vi "Update Controller State.vi"(8 "error in (no error)":errorcluster, 11 "Car Wash Controller in":refnum<class "Car Wash Controller.lvclass">) -> (0 "error out":errorcluster, 3 "Car Wash Controller out":refnum<class "Car Wash Controller.lvclass">)   [LabVIEW 2019, in "Car Wash Controller.lvlib" / "Car Wash Controller.lvclass"]
uses:
  Car Wash Controller.lvclass
  <vilib>/ActorFramework/Actor/Actor.lvclass
  Sim Configuration Database Actor/Sim Configuration Database Actor Messages/Read Record Msg/Read Record Msg.lvclass
  Sim Configuration Database Actor/Sim Configuration Database Actor Messages/Select DB Msg/Select DB Msg.lvclass
  Sim Configuration Database Actor/Sim Configuration Database Actor Messages/Write Record Msg/Write Record Msg.lvclass
  Sim Configuration Database Actor/Sim Configuration Database Actor/Database Type.ctl
  Sim Configuration Database Actor/Sim Configuration Database Actor/Sim Configuration Database Actor.lvclass
  Sim Entry Console Actor/Sim Entry Console Actor Messages/Enable Wash Steps Msg/Enable Wash Steps Msg.lvclass
  Sim Entry Console Actor/Sim Entry Console Actor Messages/Enable Start Msg/Enable Start Msg.lvclass
  Sim Wash Display Console/Sim Wash Display Console Messages/Write Remaining timing Msg/Write Remaining timing Msg.lvclass
  Sim Wash Display Console/Sim Wash Display Console Messages/Write Vehicle Out of Position Msg/Write Vehicle Out of Position Msg.lvclass
  Sim Wash Display Console/Sim Wash Display Console Messages/Write Wash Step Indicator Msg/Write Wash Step Indicator Msg.lvclass
  Sim Wash Display Console/Sim Wash Display Console Messages/Write Wash Entry Msg/Write Wash Entry Msg.lvclass
  Wash Steps.ctl
  Vehicle Position Simulation Actor/Vehicle Position Simulation Actor Messages/Write Vehicle Position Msg/Write Vehicle Position Msg.lvclass
  <vilib>/ActorFramework/Message Enqueuer/Message Enqueuer.lvclass
  Car Wash Controller Messages/Set Vehicle Position Msg/Set Vehicle Position Msg.lvclass
  Car Wash Controller Messages/Set Entry Position Msg/Set Entry Position Msg.lvclass
  Vehicle Position Simulation Actor/Car Wash Controller/Station -Enum.ctl
  Vehicle Position Simulation Actor/Car Wash Controller/Vehicle Position Simulation Actor.lvclass
  Car Wash Controller Messages/Set State Msg/Set State Msg.lvclass
  States -Enum.ctl
  C:/Program Files (x86)/National Instruments/LabVIEW 2019/vi.lib/ActorFramework/Actor/Actor.lvclass
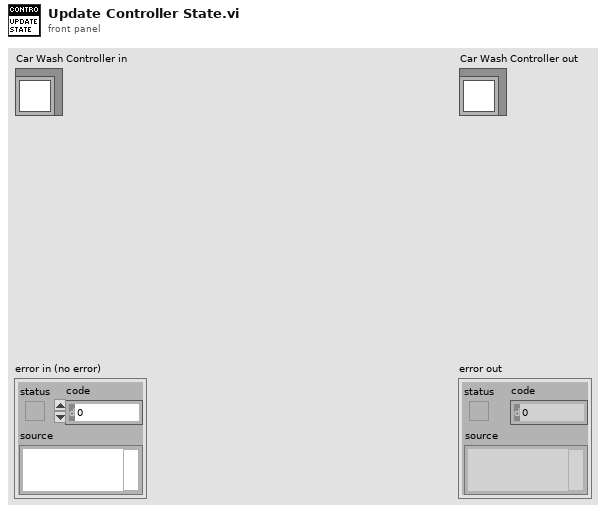
[diagram p1: front panel]
types:
  T1 = typedef "Car Wash Controller.lvlib/Car Wash Controller.lvclass/Wash Steps.ctl" = cluster{"Under Body Wash":bool, "Bug Remover":bool, "Pre-Soak":bool, "High Pressure Wash (Default)":bool, "Low Pressure Wax":bool, "Spot Free Rinse":bool, "Tire Shine Foam":bool, "Air Dry":bool}
  T2 = enum8{"Enabled", "Disabled", "Disabled and Grayed Out"}
  T3 = typedef "Sim Configuration Database Actor.lvlib/Sim Configuration Database Actor.lvclass/Database Type.ctl" = enum16{"Default", "Client"}
  T4 = typedef "Car Wash Controller.lvlib/Car Wash Controller.lvclass/States -Enum.ctl" = enum16{"Inital", "Wait for Start", "Start", "Wait for Vehicle Position", "Wash Step Execution", "Wash Step/Cycle Completion", "Wash Exit", "Wash Abort/Terminate State"}
  T5 = typedef "Vehicle Position Sinmulation Actor.lvlib/Vehicle Position Simulation Actor.lvclass/Station -Enum.ctl" = enum16{"Entry", "Station1", "Station2", "Station3", "Exit"}
  T6 = typedef "Sim Configuration Database Actor.lvlib/Sim Configuration Database Actor.lvclass/Record.ctl" = cluster{"Wash Step":string, "Step Duration":dbl, "Station":T5}
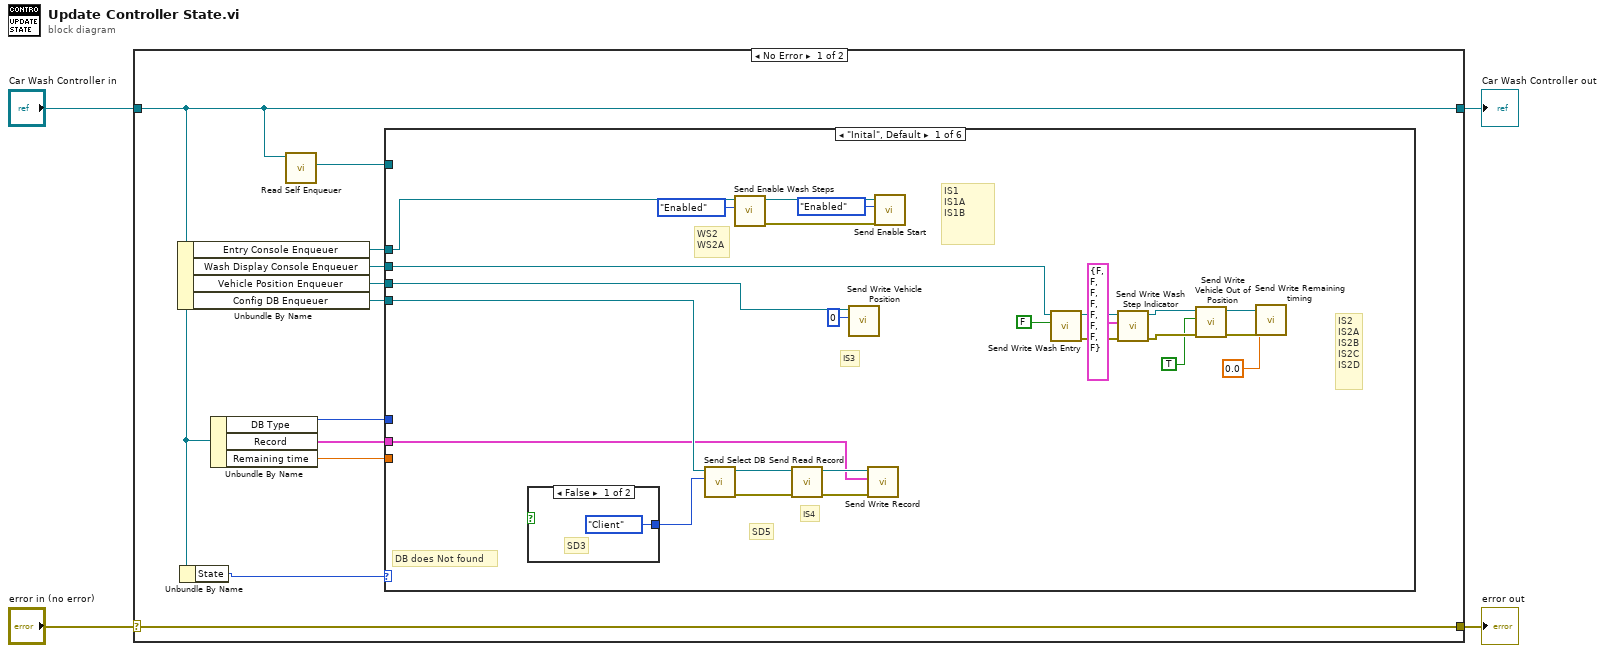
[diagram p0: block diagram]
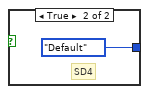
[diagram p2: hidden frame]
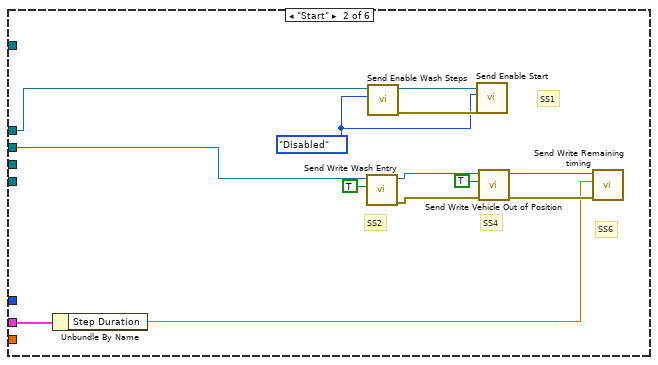
[diagram p3: hidden frame]
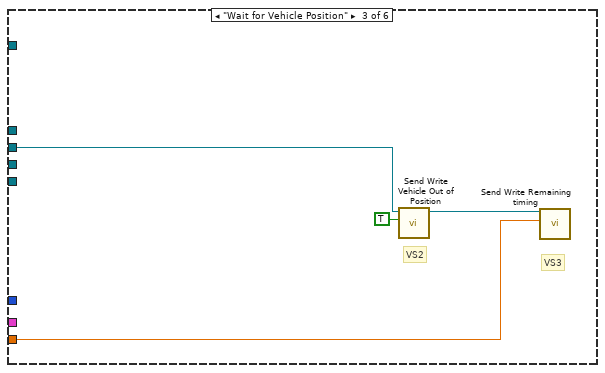
[diagram p4: hidden frame]
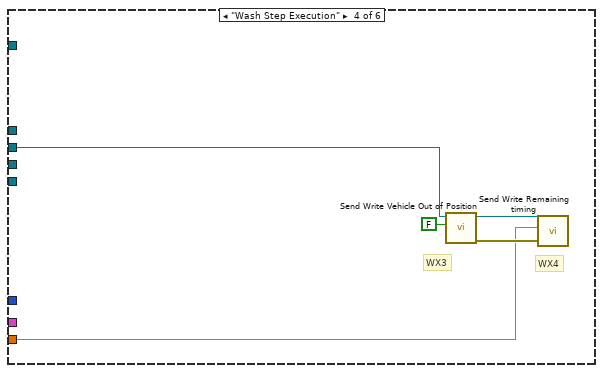
[diagram p5: hidden frame]
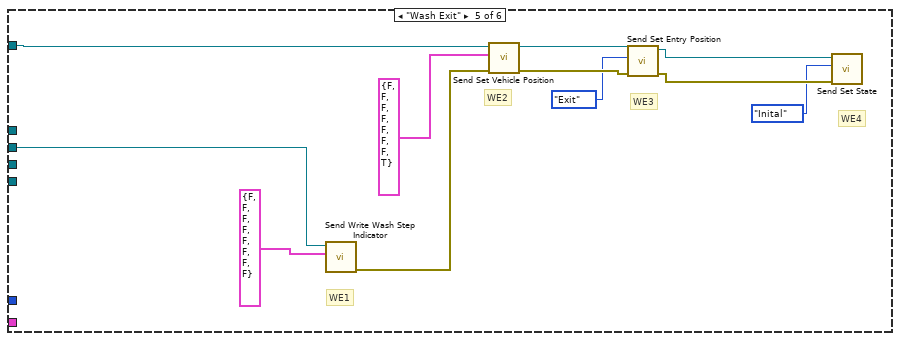
[diagram p6: hidden frame]
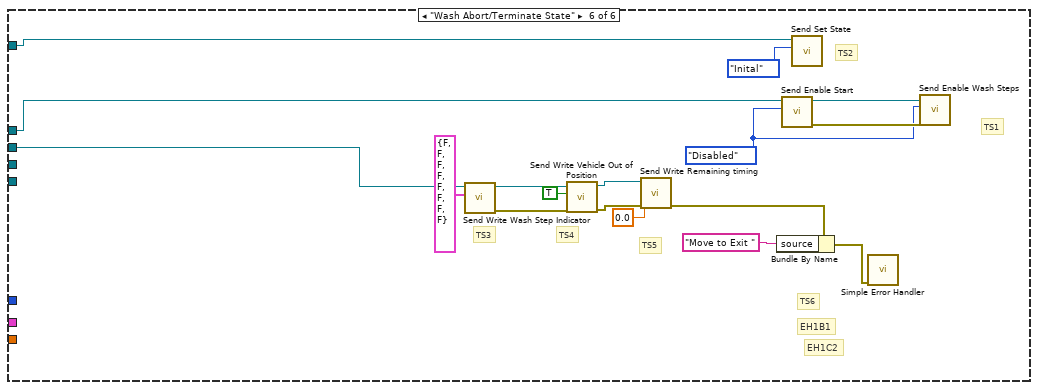
[diagram p7: hidden frame]
diagram:
  n1 = case shown="No Error" "error in (no error)" {
    selector: "error in (no error)" -> [w15 w94]
    tunnel: [w15 w94] -> w3
    tunnel: [w8 w93] -> w1
    tunnel: "Car Wash Controller in" -> [w8 w93]
    frame No Error {
      n2 = Unbundle By Name(w8) -> ("Entry Console Enqueuer"=w13:refnum<class "Message Enqueuer.lvclass">, "Wash Display Console Enqueuer"=w12:refnum<class "Message Enqueuer.lvclass">, "Vehicle Position Enqueuer"=w11:refnum<class "Message Enqueuer.lvclass">, "Config DB Enqueuer"=w10:refnum<class "Message Enqueuer.lvclass">)
      n3 = Unbundle By Name(w8) -> ("State"=w14:T4)
      n4 = Unbundle By Name(w8) -> ("DB Type"=w6:T3, "Record"=w7:T6, "Remaining time"=w5:dbl)
      n5 = call <vilib>:"Read Self Enqueuer.vi"("Actor"=w8) -> ("Self Enqueuer"=w9:refnum<class "Message Enqueuer.lvclass">)  [unwired: 10 in]
      n6 = case shown="\"Inital\", Default" w14 {
        tunnel: w13 -> [w33 w53 _ _ _ w90]
        tunnel: w12 -> [w27 w51 w58 w63 w74 w86]
        tunnel: w11 -> [w17 _ _ _ _ _]
        tunnel: w10 -> [w36 _ _ _ _ _]
        tunnel: w9 -> [_ _ _ _ w73 w88]
        tunnel: w7 -> [w34 w44 _ _ _ _]
        tunnel: w6 -> [_ _ _ _ _ _]
        tunnel: w5 -> [_ _ w56 w60 _ _]
        frame "Inital", Default {
          # "WS2\nWS2A"
          # "IS4"
          # "IS3"
          # "IS2\nIS2A\nIS2B\nIS2C\nIS2D"
          # "IS1\nIS1A\nIS1B"
          # "SD5"
          # "DB does Not found"
          n7 = case shown="False" {
            selector: _ -> [_ _]
            tunnel: [Database_Type."Client" ("DB Type") Database_Type."Default" ("DB Type")] -> w35
            frame False {
              # "SD3"
            }
            frame True {
              # "SD4"
            }
          }
          n8 = call "Send Select DB.vi"("DB Type"=w35, "Message Enqueuer"=w36) -> ("error out"=w40:errorcluster, "Message Enqueuer out"=w38:refnum<class "Message Enqueuer.lvclass">)  [unwired: 8 in]
          n9 = call "Send Enable Wash Steps.vi"("Disabled"=T2."Enabled", "Message Enqueuer"=w33) -> ("error out"=w30:errorcluster, "Message Enqueuer out"=w31:refnum<class "Message Enqueuer.lvclass">)  [unwired: 8 in]
          n10 = call "Send Read Record.vi"("error in (no error)"=w40, "Message Enqueuer"=w38) -> ("error out"=w39:errorcluster, "Message Enqueuer out"=w37:refnum<class "Message Enqueuer.lvclass">)  [unwired: 8 in]
          n11 = call "Send Write Vehicle Position.vi"("Vehicle Position Simulation"=u8 0, "Message Enqueuer"=w17) -> ()  [unwired: 8 in, 2 out]
          n12 = call "Send Write Record.vi"("error in (no error)"=w39, "Record"=w34, "Message Enqueuer"=w37) -> ()  [unwired: 7 in, 2 out]
          n13 = call "Send Enable Start.vi"("error in (no error)"=w30, "Disabled"=T2."Enabled", "Message Enqueuer"=w31) -> ()  [unwired: 7 in, 2 out]
          n14 = call "Send Write Wash Entry.vi"("Wash Entry"=FALSE, "Message Enqueuer"=w27) -> ("error out"=w28:errorcluster, "Message Enqueuer out"=w24:refnum<class "Message Enqueuer.lvclass">)  [unwired: 8 in]
          n15 = call "Send Write Wash Step Indicator.vi"("error in (no error)"=w28, "Wash Steps"=T1 {"Under Body Wash"=FALSE, "Bug Remover"=FALSE, "Pre-Soak"=FALSE, "High Pressure Wash (Default)"=FALSE, "Low Pressure Wax"=FALSE, "Spot Free Rinse"=FALSE, "Tire Shine Foam"=FALSE, "Air Dry"=FALSE}, "Message Enqueuer"=w24) -> ("error out"=w26:errorcluster, "Message Enqueuer out"=w23:refnum<class "Message Enqueuer.lvclass">)  [unwired: 7 in]
          n16 = call "Send Write Vehicle Out of Position.vi"("error in (no error)"=w26, "Vehicle Out of Position"=TRUE, "Message Enqueuer"=w23) -> ("error out"=w25:errorcluster, "Message Enqueuer out"=w22:refnum<class "Message Enqueuer.lvclass">)  [unwired: 7 in]
          n17 = call "Send Write Remaining timing.vi"("error in (no error)"=w25, "Timing Remaining"=0.0, "Message Enqueuer"=w22) -> ()  [unwired: 7 in, 2 out]
        }
        frame "Start" {
          w52 = T2."Disabled" ("Disabled")
          # "SS4"
          # "SS6"
          # "SS2"
          # "SS1"
          n18 = Unbundle By Name(w44) -> ("Step Duration"=w43:dbl)
          n19 = call "Send Write Wash Entry.vi"("Wash Entry"=TRUE, "Message Enqueuer"=w51) -> ("error out"=w49:errorcluster, "Message Enqueuer out"=w48:refnum<class "Message Enqueuer.lvclass">)  [unwired: 8 in]
          n20 = call "Send Enable Wash Steps.vi"("Disabled"=w52, "Message Enqueuer"=w53) -> ("error out"=w55:errorcluster, "Message Enqueuer out"=w54:refnum<class "Message Enqueuer.lvclass">)  [unwired: 8 in]
          n21 = call "Send Enable Start.vi"("error in (no error)"=w55, "Disabled"=w52, "Message Enqueuer"=w54) -> ()  [unwired: 7 in, 2 out]
          n22 = call "Send Write Vehicle Out of Position.vi"("error in (no error)"=w49, "Vehicle Out of Position"=TRUE, "Message Enqueuer"=w48) -> ("error out"=w46:errorcluster, "Message Enqueuer out"=w45:refnum<class "Message Enqueuer.lvclass">)  [unwired: 7 in]
          n23 = call "Send Write Remaining timing.vi"("error in (no error)"=w46, "Timing Remaining"=w43, "Message Enqueuer"=w45) -> ()  [unwired: 7 in, 2 out]
        }
        frame "Wait for Vehicle Position" {
          # "VS3"
          # "VS2"
          n24 = call "Send Write Vehicle Out of Position.vi"("Vehicle Out of Position"=TRUE, "Message Enqueuer"=w58) -> ("Message Enqueuer out"=w57:refnum<class "Message Enqueuer.lvclass">)  [unwired: 8 in, 1 out]
          n25 = call "Send Write Remaining timing.vi"("Timing Remaining"=w56, "Message Enqueuer"=w57) -> ()  [unwired: 8 in, 2 out]
        }
        frame "Wash Step Execution" {
          # "WX4"
          # "WX3"
          n26 = call "Send Write Vehicle Out of Position.vi"("Vehicle Out of Position"=FALSE, "Message Enqueuer"=w63) -> ("error out"=w61:errorcluster, "Message Enqueuer out"=w62:refnum<class "Message Enqueuer.lvclass">)  [unwired: 8 in]
          n27 = call "Send Write Remaining timing.vi"("error in (no error)"=w61, "Timing Remaining"=w60, "Message Enqueuer"=w62) -> ()  [unwired: 7 in, 2 out]
        }
        frame "Wash Exit" {
          # "WE4"
          # "WE3"
          # "WE2"
          # "WE1"
          n28 = call "Send Write Wash Step Indicator.vi"("Wash Steps"=T1 {"Under Body Wash"=FALSE, "Bug Remover"=FALSE, "Pre-Soak"=FALSE, "High Pressure Wash (Default)"=FALSE, "Low Pressure Wax"=FALSE, "Spot Free Rinse"=FALSE, "Tire Shine Foam"=FALSE, "Air Dry"=FALSE}, "Message Enqueuer"=w74) -> ("error out"=w72:errorcluster)  [unwired: 8 in, 1 out]
          n29 = call "Send Set Vehicle Position.vi"("error in (no error)"=w72, "Wash Steps"=T1 {"Under Body Wash"=FALSE, "Bug Remover"=FALSE, "Pre-Soak"=FALSE, "High Pressure Wash (Default)"=FALSE, "Low Pressure Wax"=FALSE, "Spot Free Rinse"=FALSE, "Tire Shine Foam"=FALSE, "Air Dry"=TRUE}, "Message Enqueuer"=w73) -> ("error out"=w70:errorcluster, "Message Enqueuer out"=w69:refnum<class "Message Enqueuer.lvclass">)  [unwired: 7 in]
          n30 = call "Send Set Entry Position.vi"("error in (no error)"=w70, "Station"=Station_-Enum."Exit", "Message Enqueuer"=w69) -> ("error out"=w66:errorcluster, "Message Enqueuer out"=w67:refnum<class "Message Enqueuer.lvclass">)  [unwired: 7 in]
          n31 = call "Send Set State.vi"("error in (no error)"=w66, "State"=States_-Enum."Inital", "Message Enqueuer"=w67) -> ()  [unwired: 7 in, 2 out]
        }
        frame "Wash Abort/Terminate State" {
          w89 = T2."Disabled" ("Disabled")
          # "EH1C2"
          # "EH1B1"
          # "TS6"
          # "TS5"
          # "TS4"
          # "TS3"
          # "TS2"
          # "TS1"
          n32 = call "Send Write Wash Step Indicator.vi"("Wash Steps"=T1 {"Under Body Wash"=FALSE, "Bug Remover"=FALSE, "Pre-Soak"=FALSE, "High Pressure Wash (Default)"=FALSE, "Low Pressure Wax"=FALSE, "Spot Free Rinse"=FALSE, "Tire Shine Foam"=FALSE, "Air Dry"=FALSE}, "Message Enqueuer"=w86) -> ("error out"=w83:errorcluster, "Message Enqueuer out"=w84:refnum<class "Message Enqueuer.lvclass">)  [unwired: 8 in]
          n33 = call "Send Write Vehicle Out of Position.vi"("error in (no error)"=w83, "Vehicle Out of Position"=TRUE, "Message Enqueuer"=w84) -> ("error out"=w80:errorcluster, "Message Enqueuer out"=w81:refnum<class "Message Enqueuer.lvclass">)  [unwired: 7 in]
          n34 = call "Send Write Remaining timing.vi"("error in (no error)"=w80, "Timing Remaining"=0.0, "Message Enqueuer"=w81) -> ("error out"=w78:errorcluster)  [unwired: 7 in, 1 out]
          n35 = Bundle By Name(cluster=w78, "source"="Move to Exit ") -> (w76:errorcluster)
          n36 = call "Send Enable Start.vi"("Disabled"=w89, "Message Enqueuer"=w90) -> ("error out"=w91:errorcluster, "Message Enqueuer out"=w92:refnum<class "Message Enqueuer.lvclass">)  [unwired: 8 in]
          n37 = call "Send Set State.vi"("State"=States_-Enum."Inital", "Message Enqueuer"=w88) -> ()  [unwired: 8 in, 2 out]
          n38 = call <vilib>:"Simple Error Handler.vi"("error in (no error)"=w76) -> ()  [unwired: 4 in, 5 out]
          n39 = call "Send Enable Wash Steps.vi"("error in (no error)"=w91, "Disabled"=w89, "Message Enqueuer"=w92) -> ()  [unwired: 7 in, 2 out]
        }
      }
    }
    frame Error {
    }
  }
  "error out" <- w3
  "Car Wash Controller out" <- w1
